vi "Periodic trigger ms.vi"(6 "Reset (false)":bool, 7 "Period ms":i32=100 min=-1 max=604800000 step=1) -> (3 "Trigger":bool)   [LabVIEW 2021, in "MatS Libs.lvlib"]
doc: "Real-time periodic trigger, synchronized with Tick Count. Instances with the same period will trigger at the same time. It does not wait, but has to be regulary checked in intervals much shorter than its period.\n<B>Period ms</B> - Can be set from -1 ms to 604 800 000 ms (1 week). Resets counter when changed.\n<B>Reset</B> - to manualy reset counter."
uses:
  <userlib>/MatS Libs/MatS Libs.lvlib
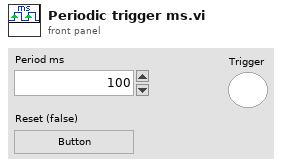
[diagram p1: front panel]
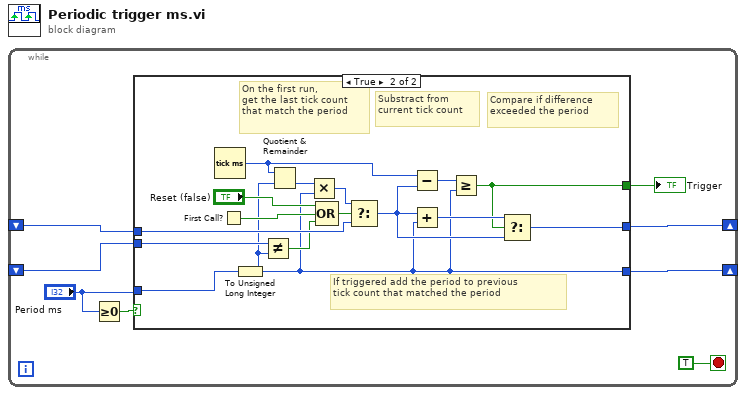
[diagram p0: block diagram]
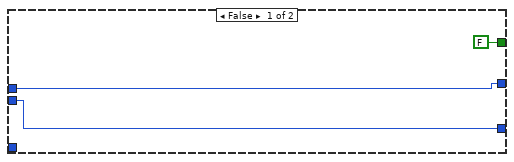
[diagram p2: hidden frame]
diagram:
  n1 = while {
    shift-right: [w7] -> _
    shift-left: _ -> [w8]
    shift-right: [w4] -> _
    shift-left: _ -> [w5]
    stop <- TRUE stop-if-true
    n2 = Greater Or Equal To 0?(x="Period ms") -> (x >= 0?=w3:bool)
    n3 = case shown="True" w3 {
      tunnel: w8 -> [w11 w27]
      tunnel: [w11 w26] -> w7
      tunnel: "Period ms" -> [_ w16]
      tunnel: w5 -> [w10 w15]
      tunnel: [w10 w13] -> w4
      tunnel: [FALSE w12] -> w1
      frame False {
      }
      frame True {
        # "If triggered add the period to previous \ntick count that matched the period"
        # "Compare if difference\nexceeded the period"
        # "Substract from\ncurrent tick count"
        # "On the first run,\nget the last tick count\nthat match the period"
        n4 = Tick Count (ms)() -> (millisecond timer value=w21:u32)
        n5 = First Call?() -> (First Call?: T/F=w24:bool)
        n6 = To Unsigned Long Integer(number=w16) -> (unsigned 32bit integer=w13:u32)
        n7 = Not Equal?(x=w15, y=w13) -> (x != y?=w14:bool)
        n8 = Quotient & Remainder(x=w21, y=w13) -> (floor(x/y)=w20:u32)  [unwired: 1 out]
        n9 = Multiply(x=w20, y=w13) -> (x*y=w19:u32)
        n10 = Compound Arithmetic op=OR("Reset (false)", w24, w14) -> (w18:bool)
        n11 = Select(t=w19, s=w18, f=w27) -> (s? t:f=w23:u32)
        n12 = Subtract(x=w21, y=w23) -> (x-y=w25:u32)
        n13 = Add(x=w23, y=w13) -> (x+y=w22:u32)
        n14 = Greater Or Equal?(x=w25, y=w13) -> (x >= y?=w12:bool)
        n15 = Select(t=w22, s=w12, f=w23) -> (s? t:f=w26:u32)
      }
    }
    "Trigger" <- w1
  }
